vi "TrajDilation.vi"(7 "Length":i32, 11 "TrajBeforeDilation":dbl[][](array[numeric])) -> (3 "TrajAfterDilation":dbl[][](array[numeric]))   [LabVIEW 2015, in "ForceField.lvclass"]
uses:
  ForceField.lvclass
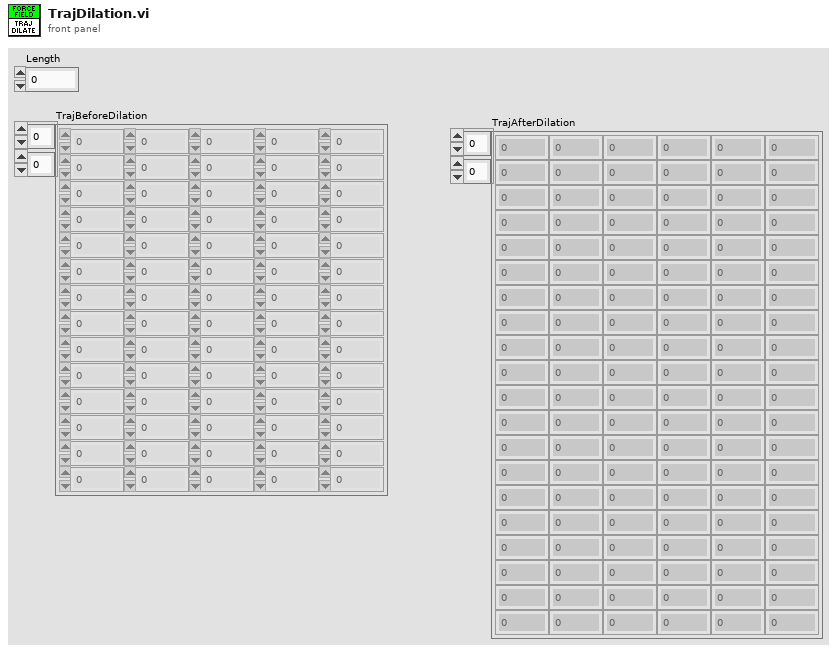
[diagram p1: front panel]
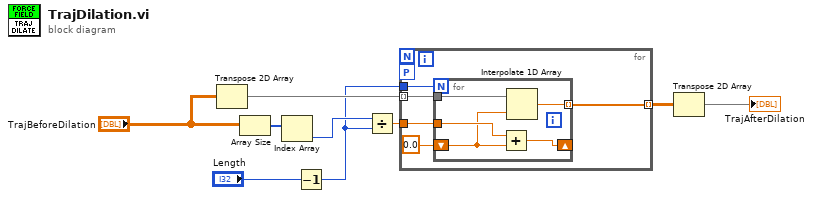
[diagram p0: block diagram]
diagram:
  n1 = Transpose 2D Array(2D array="TrajBeforeDilation") -> (transposed array=w5:dbl[][])
  n2 = Array Size(array="TrajBeforeDilation") -> (size(s)=w7:i32[])
  n3 = Index Array(array=w7) -> (element=w2:i32)  [unwired: 1 in]
  n4 = Decrement(x="Length") -> (x-1=w1:i32)
  n5 = Divide(x=w2, y=w1) -> (x/y=w8:dbl)
  n6 = for {
    tunnel: w5 -> [w14] mode=indexing
    workers-P: _ -> [_]
    tunnel: w8 -> [w11]
    tunnel: [w13] -> w9 mode=indexing
    tunnel: w1 -> [w10]
    n7 = for {
      N: w10 -> [_]
      tunnel: w14 -> [w19]
      tunnel: [w17] -> w13 mode=indexing
      shift-right: [w18] -> _
      shift-left: 0.0 ("index") -> [w15]
      tunnel: w11 -> [w16]
      n8 = Add(x=w16, y=w15) -> (x+y=w18:dbl)
      n9 = Interpolate 1D Array(1:w15, 2:w19) -> (0:w17:dbl)
    }
  }
  n10 = Transpose 2D Array(2D array=w9) -> (transposed array=→"TrajAfterDilation":dbl[][])
